vi "TestForceGraph 3.vi"() -> ()   [LabVIEW 2017]
panel:
  in  "SpectConfigAuto":T1
  in  "FirstTouch 2":T2={"FirstPeakforce"=2.0, "F_LengthView"=20, "A_LengthView "=20} {"FirstPeakforce" format="%#_13g"}
  in  "Show Name Auto":cluster{"ShowArrow":bool, "Alias":bool}
  in  "SpectConfigMan":T3
  in  "FirstTouch":T2={"FirstPeakforce"=0.2, "F_LengthView"=0, "A_LengthView "=0} {"FirstPeakforce" format="%#_13g"}
  in  "ShowName":cluster{"ShowArrow":bool, "Alias":bool}
  out "ResultUp":bool
  out "ResultDown":bool
  out "IndexFile":i32
  in  "Auto Change File":bool
  out "folder names":string[](array[string])
  in  "Full Angle Space":dbl=6.0
  in  "Full Angle Tolerance":dbl=3.0
  in  "Peak Force Tolerance":dbl=3.0
  in  "Peak Force Space":dbl=4.0
  in  "Force Annotation":bool=TRUE
  in  "Expand":bool=TRUE
  in  "Auto":bool
  in  "First Touch":bool
  in  "Path":path
  out "Filenames":string[](array[string])
  in  "FileType":string(combo)="DL"
  out "Graph":cluster{"Y":dbl[], "Y":dbl[]}[](graph)
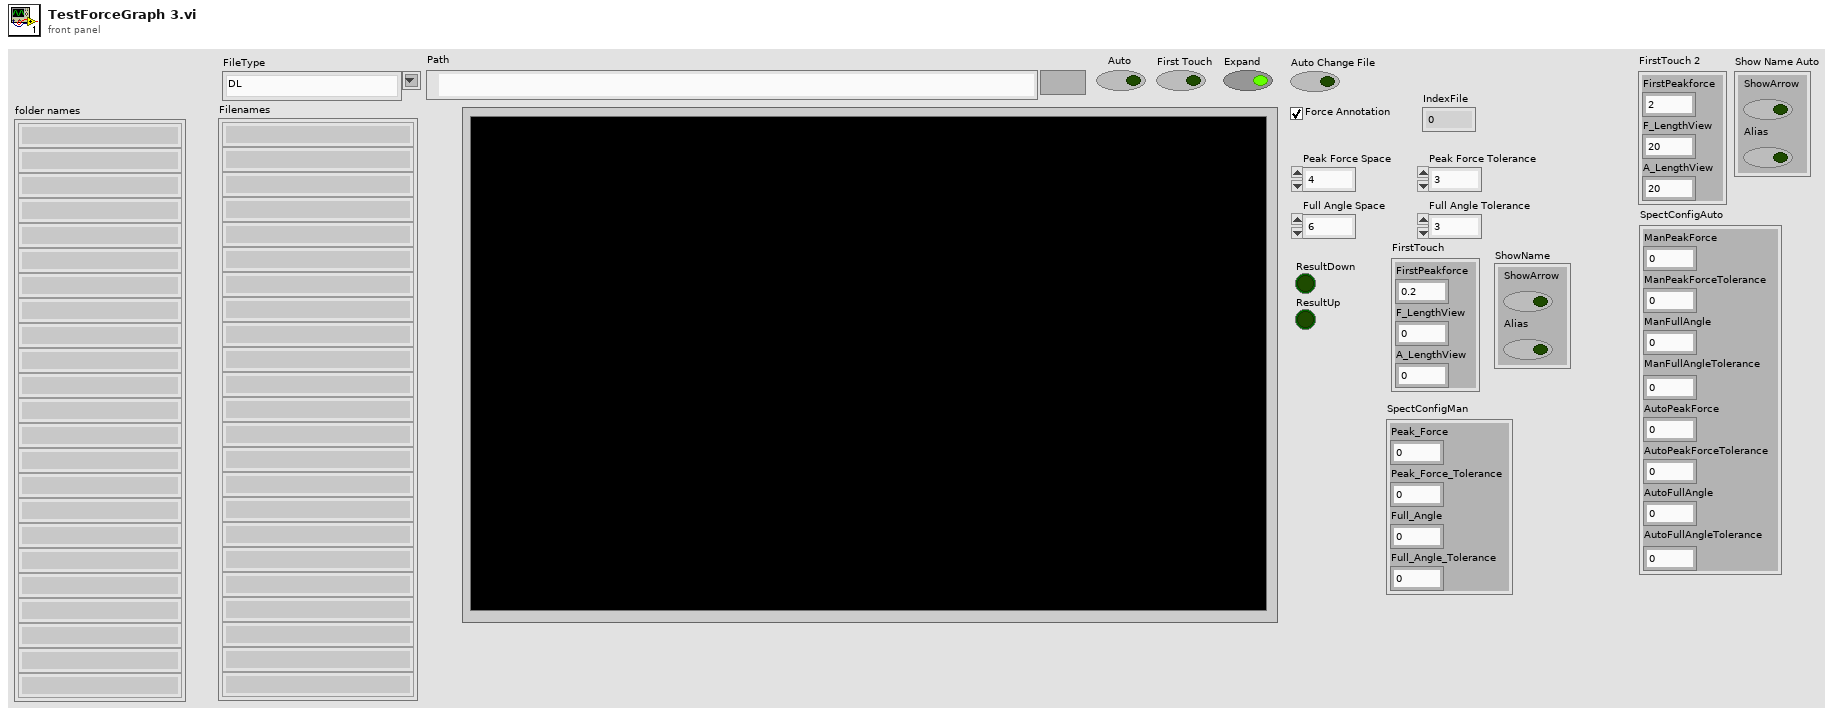
[diagram p1: front panel]
types:
  T1 = cluster{"ManPeakForce":dbl, "ManPeakForceTolerance":dbl, "ManFullAngle":dbl, "ManFullAngleTolerance":dbl, "AutoPeakForce":dbl, "AutoPeakForceTolerance":dbl, "AutoFullAngle":dbl, "AutoFullAngleTolerance":dbl}
  T2 = cluster{"FirstPeakforce":dbl, "F_LengthView":i32, "A_LengthView ":i32}
  T3 = cluster{"Peak_Force":dbl, "Peak_Force_Tolerance":dbl, "Full_Angle":dbl, "Full_Angle_Tolerance":dbl}
  T4 = cluster{"DownMax":u16, "DownMin":u16, "UpMax":u16, "UpMin":u16}
  T5 = cluster{"Angle Data":dbl[], "Force Data":dbl[], "Volt Data 1":dbl[], "Volt Data 2":dbl[]}
  T6 = cluster{"Angle Data":dbl[], "Force Data 1":dbl[], "Force Data 2":dbl[], "Volt Data 1":dbl[], "Volt Data 2":dbl[]}
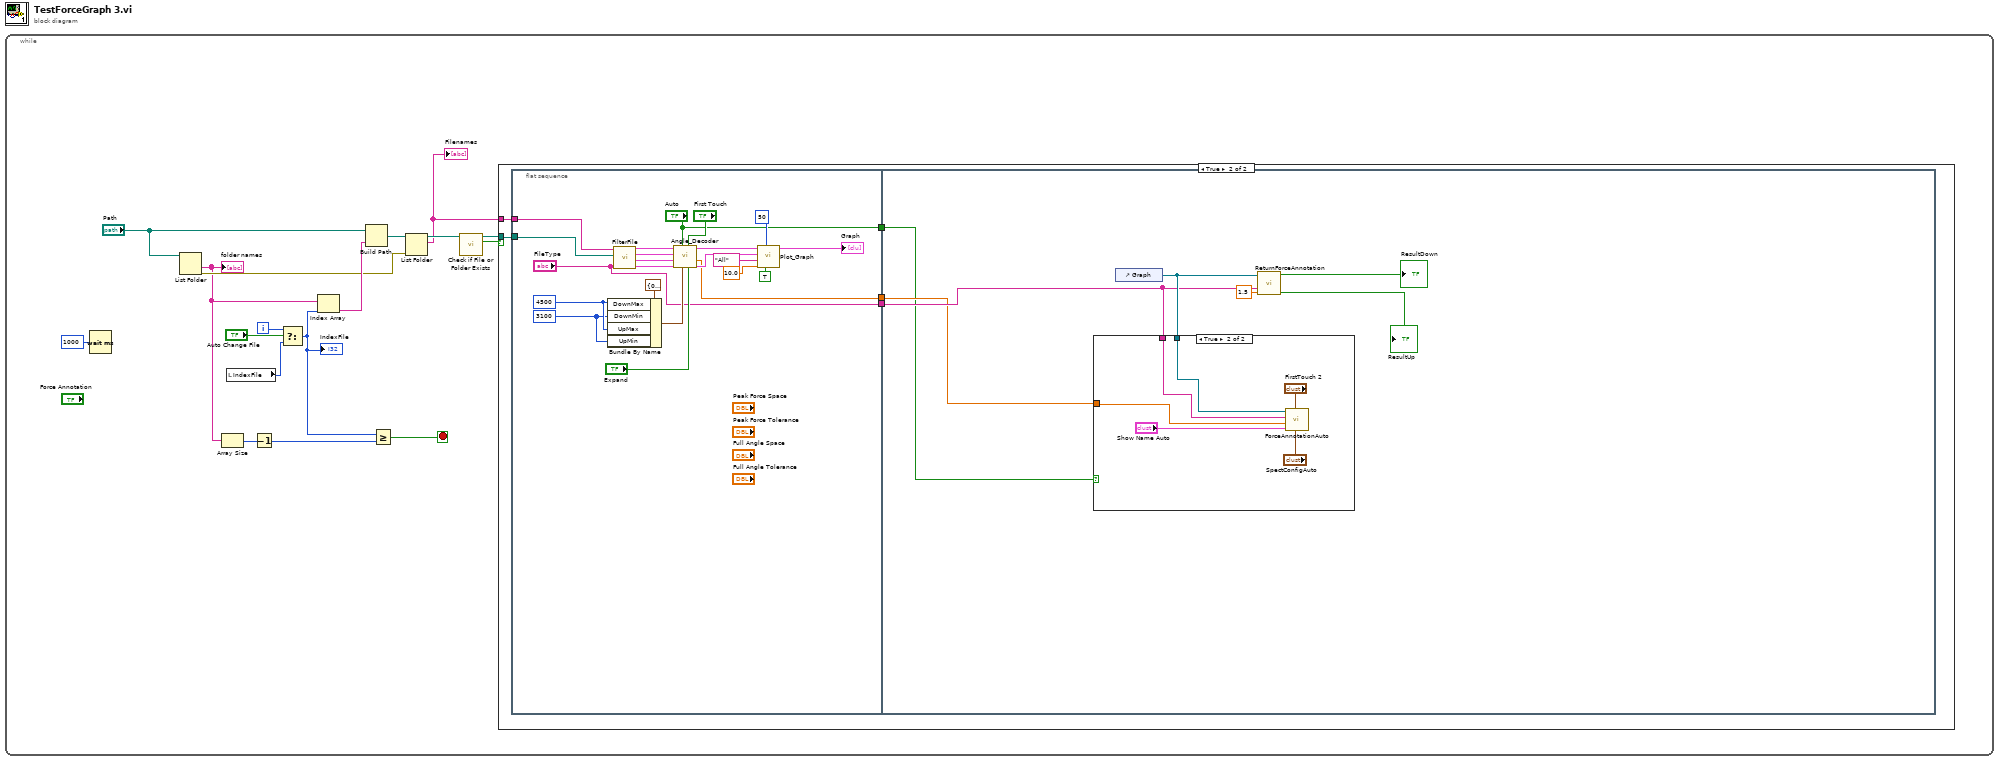
[diagram p0: block diagram]
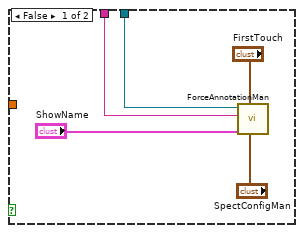
[diagram p3: hidden frame]
diagram:
  n1 = while {
    i -> [w4]
    stop <- w7 stop-if-true
    n2 = Wait (ms)(milliseconds to wait=u32 1000) -> ()  [unwired: 1 out]
    n3 = List Folder(path="Path") -> (folder names=w8:string[], error out=w11:errorcluster)  [unwired: 3 in, 2 out]
    "folder names" <- w8
    n4 = Array Size(array=w8) -> (size(s)=w6:i32)
    n5 = local read "IndexFile"() -> (w1:i32)
    n6 = Decrement(x=w6) -> (x-1=w5:i32)
    n7 = Select(t=w4, s="Auto Change File", f=w1) -> (s? t:f=w3:i32)
    "IndexFile" <- w3
    n8 = Index Array(array=w8, index=w3) -> (element=w13:string)
    n9 = Build Path(base path="Path", name or relative path=w13) -> (appended path=w12:path)
    n10 = Greater Or Equal?(x=w3, y=w5) -> (x >= y?=w7:bool)
    n11 = List Folder(path=w12, error in=w11) -> (path out=w10:path, filenames=w9:string[])  [unwired: 2 in, 2 out]
    "Filenames" <- w9
    n12 = call <vilib>:"Check if File or Folder Exists.vi"("path"=w10) -> ("file or folder exists?"=w17:bool, "dup path"=w16:path)  [unwired: 8 in, 1 out]
    n13 = case shown="True" w17 {
      tunnel: w16 -> [_ w22]
      tunnel: w9 -> [_ w19]
      frame False {
      }
      frame True {
        n14 = flat-sequence {
          tunnel: w22 -> [w37]
          tunnel: ["FileType"] -> w21
          tunnel: [w26] -> w20
          tunnel: w19 -> [w25]
          tunnel: ["Auto"] -> w18
          tunnel: w21 -> [w47]
          tunnel: w20 -> [w46]
          tunnel: w18 -> [w45]
          frame #0 {
            w30 = u16 3100
            w31 = u16 4500
            n15 = Bundle By Name(cluster=T4 {"DownMax"=0, "DownMin"=0, "UpMax"=0, "UpMin"=0} ("AngleUpDown"), "DownMax"=w31, "DownMin"=w30, "UpMax"=w31, "UpMin"=w30) -> (w38:T4)
            n16 = call "FilterFile.vi"("FileType"="FileType", "Path"=w37, "Filenames"=w25) -> ("RW_Up"=w44:T5, "FW_Up"=w35:T5, "RW_Down"=w43:T5, "FW_Down"=w36:T5)  [unwired: 3 in, 2 out]
            n17 = call "Angle_Decoder.vi"("Expand"="Expand", "Find Fist Touch"="First Touch", "AngleUpDown"=w38, "Auto/Manual"="Auto", "Analog RW Up"=w44, "Analog FW Up"=w35, "Analog RW Down"=w43, "Analog FW Down"=w36) -> ("Analog RW D/U"=w33:T6, "Last Angle"=w26:dbl, "Analog FW D/U"=w34:T6)  [unwired: 1 in]
            n18 = call "Plot_Graph.vi"("EnableSmooth"=TRUE, "FillZeroFirstSignal"=50, "VoltDevider"=10.0, "Channel"="All", "Analog RW In"=w33, "Analog FW In"=w34) -> ("XY Graph"=→"Graph":cluster{"Angle Data":dbl[], "Array":dbl[]}[])  [unwired: 5 in]
          }
          frame #1 {
            n19 = control-ref of="Graph"() -> (w48:refnum<vi>)
            n20 = case shown="True" w45 {
              tunnel: w48 -> [w53 w57]
              tunnel: w47 -> [w52 w58]
              tunnel: w46 -> [_ w59]
              frame False {
                n21 = call "ForceAnnotationMan.vi"("SpectConfig"="SpectConfigMan", "FirstTouch"="FirstTouch", "ShowName"="ShowName", "Test Name"=w52, "Graph"=w53) -> ()  [unwired: 3 in, 4 out]
              }
              frame True {
                n22 = call "ForceAnnotationAuto.vi"("SpectConfig"="SpectConfigAuto", "FirstTouch"="FirstTouch 2", "ShowName"="Show Name Auto", "LastAngle"=w59, "Test Name"=w58, "Graph"=w57) -> ()  [unwired: 2 in, 4 out]
              }
            }
            n23 = call "ReturnForceAnnotation.vi"("ReturnForce"=1.5, "Test Name"=w47, "Graph"=w48) -> ("ResultUp"=→"ResultUp":bool, "ResultDown"=→"ResultDown":bool)  [unwired: 7 in]
          }
        }
      }
    }
  }
